vi "Get Select Data.vi"(9 "Channel Tag[]":string[](array[string]), 10 "波形图":refnum<vi>) -> (2 "Data":waveform(sgl)[](array[waveform]))   [LabVIEW 2016]
uses:
  GlobleVariables/GlobleVariables.vi
  GlobleVariables/Ctrl_Sample Configure.ctl
  DataReview/Controls/Read Condition.ctl
panel:
  in  "error in":errorcluster caption="错误输入（无错误）"
  out "error out":errorcluster caption="错误输出"
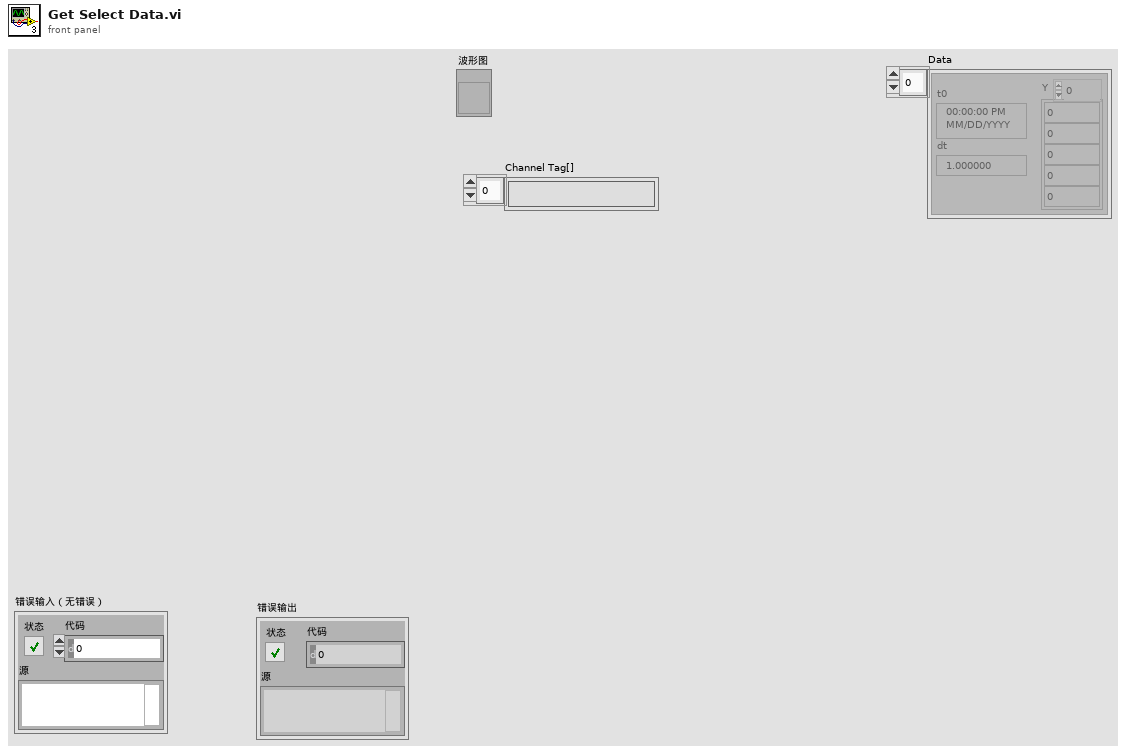
[diagram p1: front panel]
types:
  T1 = typedef "Ctrl_Sample Configure.ctl" = enum16{"Read", "Set"}
  T2 = typedef "Read Condition.ctl" = cluster{"Read Center Time":timestamp, "Read Start Time":timestamp, "Read End Time":timestamp, "Group Name":string, "Channel Names":string[]}
  T3 = typedef "ConfigureInfo.ctl" = cluster{"System":T4, "Signal[]":T5[], "Analyze Set":T6}
  T4 = typedef "System Config Information.ctl" = cluster{"测试名称":string, "存储文件夹路径":path, "存储时间间隔(min)":dbl, "采样率(HZ)":dbl, "非动态信号采样率(HZ)":dbl, "数据刷新频率(HZ)":dbl, "默认波形图个数":u8}
  T5 = typedef "Signal Information.ctl" = cluster{"Signal Type":string, "Channels Tag":string[], "Channels Name":string[], "Unit":string[], "Alarm Upper Limit":dbl[], "Alarm Lower Limit":dbl[], "Sensitivity":dbl[], "SampleRate":dbl[], "Sensor":string[], "FilterFreq":string[], "InputMode":string[], "AntiAliasingFilter":string[]}
  T6 = typedef "Analyze Set.ctl" = cluster{"FFT Set":T7, "Power Set":T8, "Shock Set":T9}
  T7 = typedef "FFT Set.ctl" = cluster{"F-W":enum16{"None", "Hanning", "Hamming", "Blackman-Harris", "Exact Blackman", "Blackman", "Flat Top", "4 Term B-Harris ", "7 Term B-Harris", "Low Sidelobe", "Force", "Exponential", "Blackman Nuttall", "Triangle", "Bartlett-Hanning", "Bohman", "Parzen", "Welch", "Kaiser", "Dolph-Chebyshev", "Gaussian"}, "F-L":dbl, "F-R":dbl}
  T8 = typedef "Power Set.ctl" = cluster{"P-W":enum16{"None", "Hanning", "Hamming", "Blackman-Harris", "Exact Blackman", "Blackman", "Flat Top", "4 Term B-Harris ", "7 Term B-Harris", "Low Sidelobe", "Force", "Exponential", "Blackman Nuttall", "Triangle", "Bartlett-Hanning", "Bohman", "Parzen", "Welch", "Kaiser", "Dolph-Chebyshev", "Gaussian"}, "P-L":dbl, "P-R":dbl}
  T9 = typedef "Shock Set.ctl" = cluster{"S-W":enum16{"None", "Hanning", "Hamming", "Blackman-Harris", "Exact Blackman", "Blackman", "Flat Top", "4 Term B-Harris ", "7 Term B-Harris", "Low Sidelobe", "Force", "Exponential", "Blackman Nuttall", "Triangle", "Bartlett-Hanning", "Bohman", "Parzen", "Welch", "Kaiser", "Dolph-Chebyshev", "Gaussian"}, "S-L":dbl, "S-R":dbl, "S-Z":dbl, "S-FFT":dbl}
  T10 = typedef "Folder Information.ctl" = cluster{"Folder Info":T11, "File Information":T12[], "Group Information":T13[]}
  T11 = typedef "TDMS File Info.ctl" = cluster{"Path":path, "Start Time":timestamp, "End Time":timestamp, "TdmsRef":refnum<k34>}
  T12 = typedef "File Information.ctl" = cluster{"File":T11, "Groups":T13[]}
  T13 = typedef "Group Information.ctl" = cluster{"Group Name":string, "Channel Names":string[], "Channel Units":string[], "dt":dbl, "Length":u64}
  T14 = typedef "File Read Parameters.ctl" = cluster{"File Parameters":T15[], "Read Condition":T2}
  T15 = typedef "Single File Read Parameter.ctl" = cluster{"File Read Information":T16, "File Information":T12}
  T16 = typedef "File Read Information.ctl" = cluster{"Zero?":bool, "Zero":i64, "Read?":bool, "Offset":i64, "Length":i64}
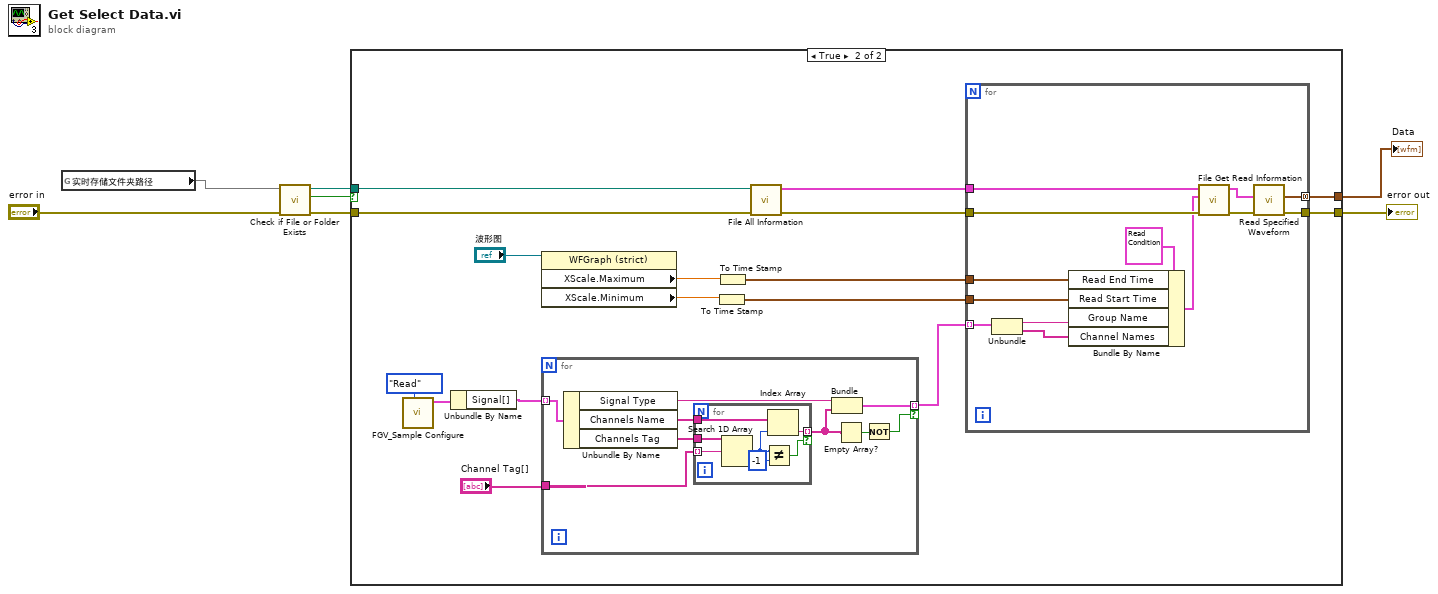
[diagram p0: block diagram]
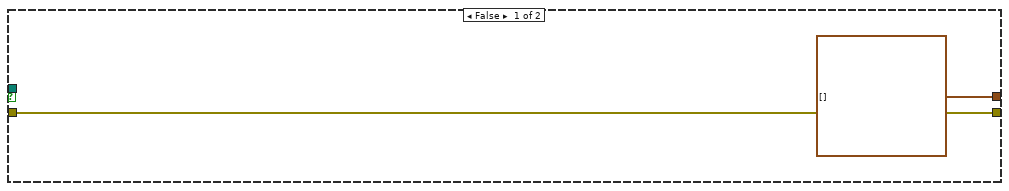
[diagram p2: hidden frame]
diagram:
  n1 = global read "GlobleVariables.vi" "实时存储文件夹路径"() -> (w2)
  n2 = call <vilib>:"Check if File or Folder Exists.vi"("error in (no error)"="error in", "path"=w2) -> ("error out"=w4:errorcluster, "file or folder exists?"=w3:bool, "dup path"=w6:path)  [unwired: 7 in]
  n3 = case shown="True" w3 {
    tunnel: [w9 w23] -> w7
    tunnel: w6 -> [_ w17]
    tunnel: w4 -> [w9 w16]
    tunnel: [waveform(sgl)[] [] ("Waveform") w15] -> w1
    frame False {
    }
    frame True {
      n4 = call "FGV_Sample Configure.vi"("Action"=Ctrl_Sample_Configure."Read") -> ("ConfigureInfo"=w20:T3)  [unwired: 9 in, 1 out]
      n5 = Unbundle By Name(w20) -> ("Signal[]"=w19:T5[])
      n6 = property on="属性节点" class="WFGraph (strict)"(reference="波形图") -> ("XScale.Maximum"=w13:dbl, "XScale.Minimum"=w12:dbl)  [unwired: 1 in, 2 out]
      n7 = for {
        tunnel: "Channel Tag[]" -> [w47]
        tunnel: w19 -> [w46] mode=indexing
        tunnel: [w42] -> w18 mode=indexing if=w39
        n8 = Unbundle By Name(w46) -> ("Signal Type"=w43:string, "Channels Name"=w44:string[], "Channels Tag"=w45:string[])
        n9 = for {
          tunnel: w47 -> [w54] mode=indexing
          tunnel: w45 -> [w53]
          tunnel: w44 -> [w52]
          tunnel: [w51] -> w41 mode=indexing if=w48
          n10 = Search 1D Array(1D array=w53, element=w54) -> (index of element=w50:i32)  [unwired: 1 in]
          n11 = Not Equal?(x=w50, y=-1) -> (x != y?=w48:bool)
          n12 = Index Array(array=w52, index=w50) -> (element=w51:string)
        }
        n13 = Bundle("Signal Type"=w43, w41) -> (w42:cluster{"Signal Type":string, string[]})  [unwired: 1 in]
        n14 = Empty Array?(array=w41) -> (empty?=w40:bool)
        n15 = Not(x=w40) -> (.not. x?=w39:bool)
      }
      n16 = To Time Stamp(1:w12) -> (0:w10:timestamp)
      n17 = To Time Stamp(1:w13) -> (0:w11:timestamp)
      n18 = call "File All Information.vi"("error in"=w16, "FoldPath"=w17) -> ("error out"=w25:errorcluster, "Folder Information"=w24:T10)  [unwired: 6 in, 2 out]
      n19 = for {
        tunnel: w25 -> [w36]
        tunnel: w24 -> [w35]
        tunnel: [w32] -> w23
        tunnel: w18 -> [w31] mode=indexing
        tunnel: w11 -> [w28]
        tunnel: w10 -> [w27]
        tunnel: [w26] -> w15 mode=concatenating
        n20 = Unbundle(w31) -> ("Signal Type"=w30:string, w29:string[])
        n21 = Bundle By Name(cluster=T2 {"Read Center Time"=timestamp(0 s since 1904-01-01), "Read Start Time"=timestamp(0 s since 1904-01-01), "Read End Time"=timestamp(0 s since 1904-01-01), "Group Name"="", "Channel Names"=[]} ("Read Condition"), "Read End Time"=w28, "Read Start Time"=w27, "Group Name"=w30, "Channel Names"=w29) -> (w33:T2)
        n22 = call "File Get Read Information.vi"("error in (no error)"=w36, "Read Condition"=w33, "Folder Information"=w35) -> ("error out"=w38:errorcluster, "Read Parameters"=w37:T14)  [unwired: 6 in, 1 out]
        n23 = call "Read Specified Waveform.vi"("error in"=w38, "Read Parameters"=w37) -> ("error out"=w32:errorcluster, "Waveform"=w26:waveform(sgl)[])  [unwired: 7 in, 1 out]
      }
    }
  }
  "Data" <- w1
  "error out" <- w7
